vi "Simulation Record Write.vi"(8 "Error In":errorcluster, 11 "simulator":T1={"configuration"={"maxTime"=5.0, "enableVisualization"=TRUE, "statechart"=path "iRobot Navigation State Machine.vi", "environment"=path "iRobot Navigation State Machine.vi", "record"=path "Simulation Record.xml", "autograde?"=TRUE, "interactive?"=FALSE, "feedback mode"=enum."debug navigation"}, "Bump Sensors"=[], "Distance Sensors"=[], "Accelerometer"=refnum, "Wall Sensor"=refnum, "Statechart\ndisplay"=refnum, "Body"=refnum, "Left Motor"=refnum, "Right Motor"=refnum, "first step?"=FALSE}) -> (0 "Error Out":errorcluster, 3 "simulator":T1={"configuration"={"maxTime"=5.0, "enableVisualization"=TRUE, "statechart"=path "iRobot Navigation State Machine.vi", "environment"=path "iRobot Navigation State Machine.vi", "record"=path "Simulation Record.xml", "autograde?"=TRUE, "interactive?"=FALSE, "feedback mode"=enum."debug navigation"}, "Bump Sensors"=[], "Distance Sensors"=[], "Accelerometer"=refnum, "Wall Sensor"=refnum, "Statechart\ndisplay"=refnum, "Body"=refnum, "Left Motor"=refnum, "Right Motor"=refnum, "first step?"=FALSE})   [LabVIEW 2013]
uses:
  Simulator.ctl
  <instrlib>/DC Motor Controller/HAIOL/DC Motor Controller.lvclass
  CyberSim interface/Simulation Configuration.ctl
  autograder/feedbackMode.ctl
  <vilib>/Utility/xml.llb/Write to XML File(string).vi
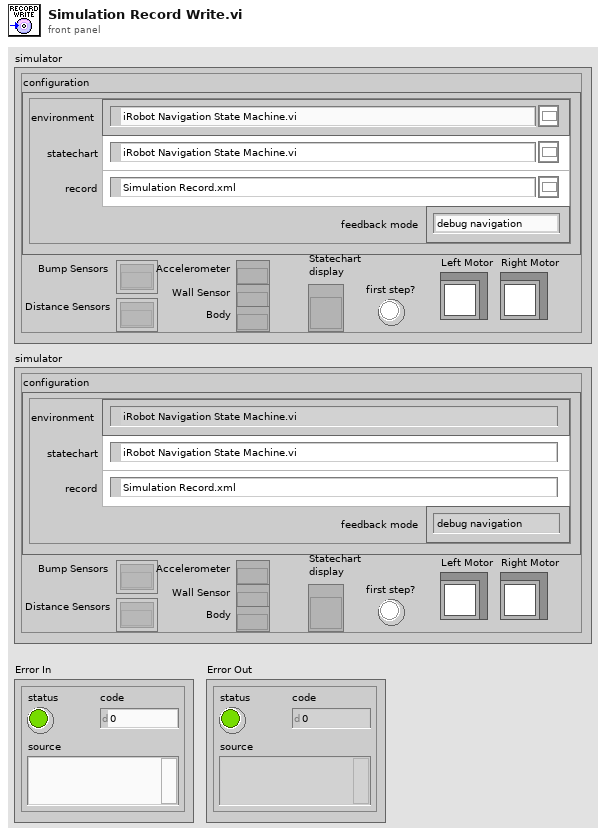
[diagram p1: front panel]
types:
  T1 = typedef "Simulator.ctl" = cluster{"configuration":T2, "Bump Sensors":refnum<k20>[], "Distance Sensors":refnum<k20>[], "Accelerometer":refnum<k20>, "Wall Sensor":refnum<k20>, "Statechart\ndisplay":refnum<vi>, "Body":refnum<k20>, "Left Motor":refnum<class "DC Motor Controller.lvclass">, "Right Motor":refnum<class "DC Motor Controller.lvclass">, "first step?":bool}
  T2 = typedef "Simulation Configuration.ctl" = cluster{"maxTime":sgl, "enableVisualization":bool, "statechart":path, "environment":path, "record":path, "autograde?":bool, "interactive?":bool, "feedback mode":T3}
  T3 = typedef "feedbackMode.ctl" = enum32{"debug navigation", "debug hill climb", "autograde navigation", "autograde hill climb"}
  T4 = typedef "Simulation Record.ctl" = cluster{"configuration":T2, "trace":T5[], "environment MD5":string, "statechart MD5":string, "record timestamp":string}
  T5 = typedef "Simulation Trace Element.ctl" = cluster{"sensors":T6, "position":T16, "orientation":T17, "Simulation Time (s)":sgl}
  T6 = typedef "Sensors.ctl" = cluster{"net distance (mm)":i32, "net angle (deg)":i32, "accelerometer":T7, "iRobot Sensors":T8, "Is Simulator?":bool}
  T7 = typedef "Accelerometer.ctl" = cluster{"x axis (g)":dbl, "y axis (g)":dbl, "z axis (g)":dbl}
  T8 = typedef "Sensor Group 6.ctl" = cluster{"Bumps + Wheel Drops":T9, "Wall":bool, "Cliff Left":bool, "Cliff Front Left":bool, "Cliff Front Right":bool, "Cliff Right":bool, "Wall Signal":u16, "Cliff Left Signal":u16, "Cliff Front Left Signal":u16, "Cliff Front Right Signal":u16, "Cliff Right Signal":u16, "Buttons":T10, "Virtual Wall":bool, "# Stream Packets":u8, "Requested Velocity (mm/s)":i16, "Requested Radius (mm)":i16, "Requested Right Wheel Velocity (mm/s)":i16, "Requested Left Wheel Velocity (mm/s)":i16, "Distance (mm)":i32, "Angle (deg)":i32, "Song Playing":bool, "Song Number":u8, "Charging State":T11, "Voltage (mV)":u16, "Current (mA)":i16, "Battery Temperature (deg C)":i8, "Battery Charge (mAh)":u16, "Battery Capacity (mAh)":u16, "Charging Sources":T12, "OI Mode":T13, "Digital Inputs":T14, "Drivers & Wheel Overcurrent":T15, "Analog Signal":u16, "Infrared":u8}
  T9 = typedef "Bumps + Wheel Drops.ctl" = cluster{"Wheeldrop Caster":bool, "Wheeldrop Left":bool, "Wheeldrop Right":bool, "Bump Left":bool, "Bump Right":bool}
  T10 = typedef "Buttons.ctl" = cluster{"Advance":bool, "Play":bool}
  T11 = typedef "Charging State.ctl" = enum16{"Not Charging", "Reconditioning Charging", "Full Charging", "Trickle Charging", "Waiting", "Charging Fault Condition"}
  T12 = typedef "Charging Sources Available.ctl" = cluster{"Internal Charger":bool, "Home Base":bool}
  T13 = typedef "OI Mode.ctl" = enum16{"Off", "Passive", "Safe", "Full"}
  T14 = typedef "Cargo Bay Digital Inputs.ctl" = cluster{"Digital Input 0":bool, "Digital Input 1":bool, "Digital Input 2":bool, "Digital Input 3":bool, "Device Detect":bool}
  T15 = typedef "Low-Side Driver + Wheel Overcurrent.ctl" = cluster{"Low-Side Driver 0":bool, "Low-Side Driver 1":bool, "Low-Side Driver 2":bool, "Left Wheel":bool, "Right Wheel":bool}
  T16 = typedef "Simulated iRobot Position.ctl" = cluster{"x (m)":sgl, "y (m)":sgl, "z (m)":sgl}
  T17 = typedef "Simulated iRobot Orientation.ctl" = cluster{"roll (deg)":sgl, "pitch (deg)":sgl, "yaw (deg)":sgl}
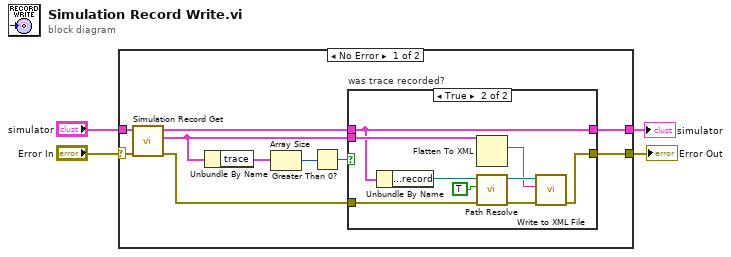
[diagram p0: block diagram]
diagram:
  n1 = case shown="No Error" "Error In" {
    selector: "Error In" -> [w5 w26]
    tunnel: [w14 w26] -> w4
    tunnel: "simulator" -> [w13 w27]
    tunnel: [w6 w27] -> w2
    frame No Error {
      n2 = call "Simulation Record Get.vi"("Error In"=w5, "simulator"=w13) -> ("Error Out"=w11:errorcluster, "record"=w10:T4, "simulator"=w12:T1)  [unwired: 7 in]
      n3 = Unbundle By Name(w10) -> ("trace"=w9:T5[])
      n4 = Array Size(array=w9) -> (size(s)=w8:i32)
      n5 = Greater Than 0?(x=w8) -> (x > 0?=w7:bool)
      n6 = case "was trace recorded?" shown="True" w7 {
        tunnel: [w16 w25] -> w14
        tunnel: w12 -> [w15 w17]
        tunnel: w11 -> [w16 w19]
        tunnel: w10 -> [_ w18]
        tunnel: [w15 w17] -> w6
        frame False {
        }
        frame True {
          n7 = Unbundle By Name(w17) -> ("configuration.record"=w20:path)
          n8 = Flatten To XML(anything=w18) -> (xml string=w21:string)
          n9 = call "Path Resolve.vi"("Error In"=w19, "create?"=TRUE, "absolute or relative path"=w20) -> ("Error Out"=w22:errorcluster, "resolved path"=w23:path)  [unwired: 7 in]
          n10 = call-poly <vilib>:"Write to XML File.vi"("error in (no error)"=w22, "XML Input"=w21, "XML File Path"=w23) -> ("error out"=w25:errorcluster)  [unwired: 6 in, 2 out]
        }
      }
    }
    frame Error {
    }
  }
  "Error Out" <- w4
  "simulator" <- w2
